vi "Connection State Callback.vi"(7 "Owner":refnum<class>, 10 "Connection State":T1, 11 "Endpoint":refnum<class "Endpoint.lvclass">) -> ()   [LabVIEW 2020, in "LV Server.lvclass"]
uses:
  LV Server.lvclass
  d6d7a9e7-92c6-4505-8a10-6da73ec66b89.vi
  e2bd68c5-6691-4f5a-b365-21e306f1d28a.vi
  Common/Message ID.ctl
  Common/Common.lvlib
  Common/Timer Init.ctl
  lv-stream/stream/Connection State.ctl
  lv-stream/stream/Stream.lvlib
  lv-msg-simple/Stream-Simple-Msg/Endpoint/Endpoint.lvclass
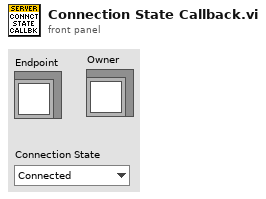
[diagram p1: front panel]
types:
  T1 = typedef "Stream.lvlib/Connection State.ctl" = enum16{"Connected", "Disconnected"}
  T2 = typedef "Common.lvlib/Timer Init.ctl" = cluster{"State":string, "Value":string}
  T3 = typedef "Common.lvlib/Message ID.ctl" = enum16{"Timer State", "Timer Value", "Timer Start", "Timer Pause", "Timer Reset", "Timer Init"}
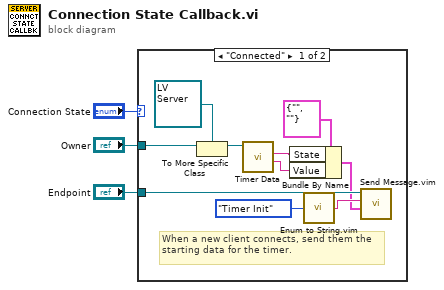
[diagram p0: block diagram]
diagram:
  n1 = case shown="\"Connected\"" "Connection State" {
    tunnel: "Owner" -> [w13 _]
    tunnel: "Endpoint" -> [w11 _]
    frame "Connected" {
      # "When a new client connects, send them the starting data for the timer."
      n2 = To More Specific Class(target class=refnum<class "LV Server.lvclass"> refnum ("LV Server.lvclass"), reference=w13) -> (specific class reference=w8:refnum<class "LV Server.lvclass">)  [unwired: 1 in, 1 out]
      n3 = call "Timer Data.vi"("LV Server in"=w8) -> ("Timer Value"=w5:string, "Timer State"=w6:string)  [unwired: 7 in, 2 out]
      n4 = Bundle By Name(cluster=T2 {"State"="", "Value"=""} ("Timer Init"), "State"=w6, "Value"=w5) -> (w4:T2)
      n5 = call "Enum to String.vim"("Enum"=Message_ID."Timer Init" ("Message ID")) -> ("Enum String"=w9:string)
      n6 = call "Send Message.vim"("Data"=w4, "ID"=w9, "Endpoint in"=w11) -> ()  [unwired: 7 in, 2 out]
    }
    frame "Disconnected" {
    }
  }
